vi "Build Self Extracting Installer.vi"(10 "Package Version":string="2.0.0.4") -> (0 "Error Out":errorcluster)   [LabVIEW 2019]
uses:
  <vilib>/AppBuilder/AB_API_Simple/Build Specification Version.ctl
  <vilib>/AppBuilder/AB_API_Simple/Set Build Specification Version (path).vi
  <vilib>/AppBuilder/AB_API_Simple/Build (path).vi
  <userlib>/LevyLab/Build Support/PostBuildSupport/PostBuildSupport.lvclass
  <vilib>/MakerHub/Toolbox/LMH-Toolbox.lvlib
  <vilib>/AppBuilder/AB_API_Simple/NI_App_Builder_API.lvlib
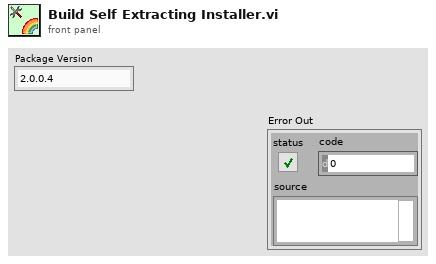
[diagram p1: front panel]
types:
  T1 = typedef "NI_App_Builder_API.lvlib/Build Specification Version.ctl" = cluster{"Major":u16, "Minor":u16, "Fix":u16, "Build":u16}
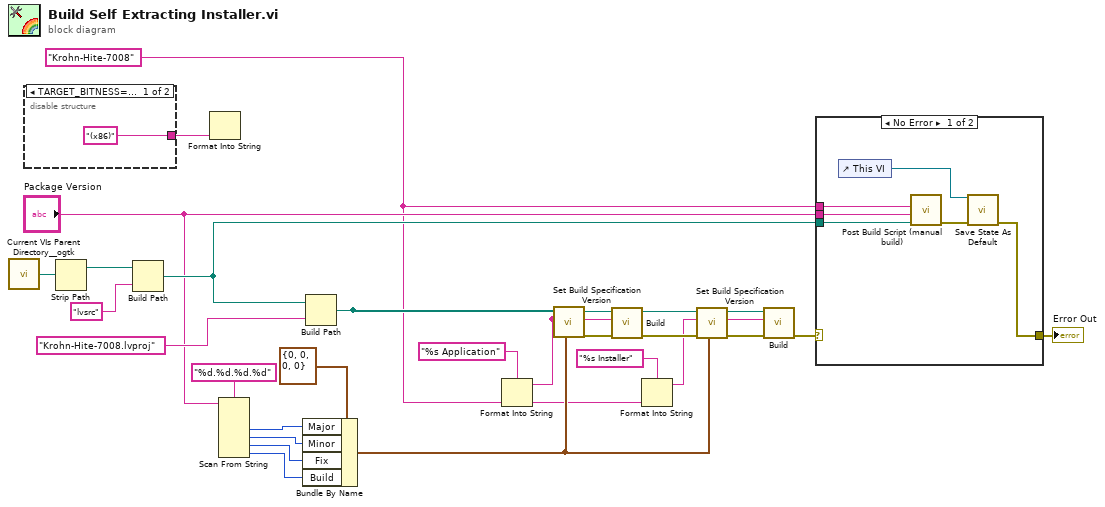
[diagram p0: block diagram]
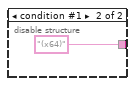
[diagram p2: hidden frame]
diagram:
  w1 = "Krohn-Hite-7008" ("Product Name")
  n1 = call <userlib>:"Current VIs Parent Directory__ogtk.vi"() -> ("Parent Directory (+ Relative)"=w25:path)  [unwired: 5 in]
  n2 = disable-structure shown="TARGET_BITNESS==32, Default" {
    disable-tunnel: ["(x86)" ("Name of build specification") "(x64)" ("Name of build specification")] -> w3
    frame condition #0 (active) {
    }
    frame condition #1 {
    }
  }
  n3 = Strip Path(path=w25) -> (stripped path=w24:path)  [unwired: 1 out]
  n4 = Build Path(base path=w24, name or relative path="lvsrc") -> (appended path=w14:path)
  n5 = Format Into String(w3) -> ()  [unwired: 3 in, 2 out]
  n6 = Scan From String(format string="%d.%d.%d.%d", input string="Package Version") -> (output 1=w19:i32, output 2=w22:i32, output 3=w18:i32, output 4=w21:i32)  [unwired: 6 in, 3 out]
  n7 = Bundle By Name(cluster=T1 {"Major"=0, "Minor"=0, "Fix"=0, "Build"=0} ("Build Specification Version"), "Major"=w19, "Minor"=w22, "Fix"=w18, "Build"=w21) -> (w16:T1)
  n8 = Build Path(base path=w14, name or relative path="Krohn-Hite-7008.lvproj") -> (appended path=w13:path)
  n9 = Format Into String(format string="%s Application" ("Name of build specification"), w1) -> (resulting string=w7:string)  [unwired: 2 in, 1 out]
  n10 = call-poly <vilib>:"Set Build Specification Version.vi"("Build Specification Version"=w16, "Name of build specification"=w7, "Path to project"=w13) -> ("error out"=w11:errorcluster)  [unwired: 8 in]
  n11 = call-poly <vilib>:"Build.vi"("error in (no error)"=w11, "Name of build specification (if empty: build all)"=w7, "Path to project"=w13) -> ("error out"=w10:errorcluster)  [unwired: 7 in, 1 out]
  n12 = Format Into String(format string="%s Installer" ("Name of build specification"), w1) -> (resulting string=w6:string)  [unwired: 2 in, 1 out]
  n13 = call-poly <vilib>:"Set Build Specification Version.vi"("Build Specification Version"=w16, "error in (no error)"=w10, "Name of build specification"=w6, "Path to project"=w13) -> ("error out"=w9:errorcluster)  [unwired: 7 in]
  n14 = call-poly <vilib>:"Build.vi"("error in (no error)"=w9, "Name of build specification (if empty: build all)"=w6, "Path to project"=w13) -> ("error out"=w4:errorcluster)  [unwired: 7 in, 1 out]
  n15 = case shown="No Error" w4 {
    selector: w4 -> [_ w34]
    tunnel: w14 -> [w31 _]
    tunnel: w1 -> [w30 _]
    tunnel: "Package Version" -> [w29 _]
    tunnel: [w28 w34] -> w2
    frame No Error {
      n16 = control-ref of="This VI"() -> (w32:refnum<vi>)
      n17 = call <userlib>:"Post Build Script (manual build).vi"("Package Source Folder"=w31, "Package Version"=w29, "Product Name"=w30) -> ("error out"=w33:errorcluster)  [unwired: 8 in]
      n18 = call <vilib>:"Save State As Default.vi"("Error In"=w33, "Target VI"=w32) -> ("Error Out"=w28:errorcluster)  [unwired: 8 in, 1 out]
    }
    frame Error {
    }
  }
  "Error Out" <- w2
